vi "Set Inhibited.vi"(8 "error in (no error)":errorcluster, 10 "Inhibit":bool, 11 "VISA resource name":refnum<visa-resource-name>="COM1") -> (0 "error out":errorcluster, 2 "query output":string, 3 "VISA resource name out":refnum<visa-resource-name>)   [LabVIEW 2017]
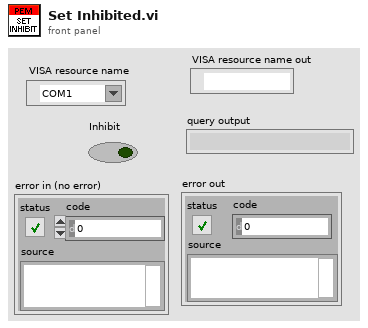
[diagram p1: front panel]
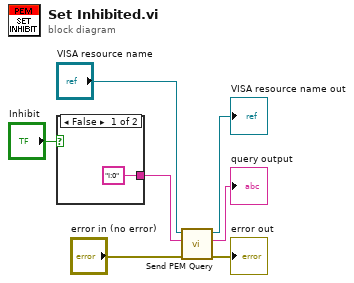
[diagram p0: block diagram]
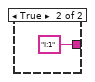
[diagram p2: hidden frame]
diagram:
  n1 = case shown="False" "Inhibit" {
    tunnel: ["I:0" ("query string") "I:1" ("query string")] -> w1
    frame False {
    }
    frame True {
    }
  }
  n2 = call "Send PEM Query.vi"("error in (no error)"="error in (no error)", "query string"=w1, "VISA resource name"="VISA resource name") -> ("error out"=→"error out":errorcluster, "query output"=→"query output":string, "VISA resource name out"=→"VISA resource name out":refnum<visa-resource-name>)  [unwired: 5 in, 1 out]
